vi "NGTS_Create Tasks from Channel Table.vi"(6 "Task Auto Cleanup?":bool, 7 "Physical Address Col (0)":i32, 8 "error in":errorcluster, 9 "Type of IO":enum16{"AI", "AO", "DI", "DO"}(ring), 11 "Channels Properties Table":string[][](array[string])) -> (0 "error out":errorcluster, 2 "List of Devices":string[](array[string]), 3 "DAQmx Task Array Out":refnum<k21>[](array[refnum]))   [LabVIEW 2018]
doc: "Creates DAQmx Tasks based on how many unique chassis IDs there are in the Channel Address column of the Channels Properties Tables. Optionally sets the Auto Cleanup of the tasks when application execution ends.\n\n2007-11 Mike Ashe\nmichael.ashe@imaginatics.net\nCell: 860-961-0876"
uses:
  <userlib>/_OpenG.lib/array/array.llb/Remove Duplicates from 1D Array (String)__ogtk.vi
panel:
  # ". . ."
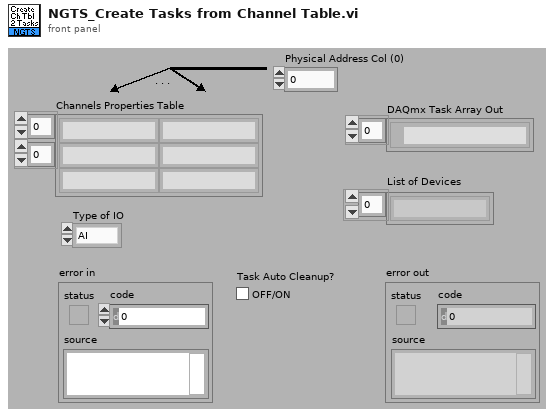
[diagram p1: front panel]
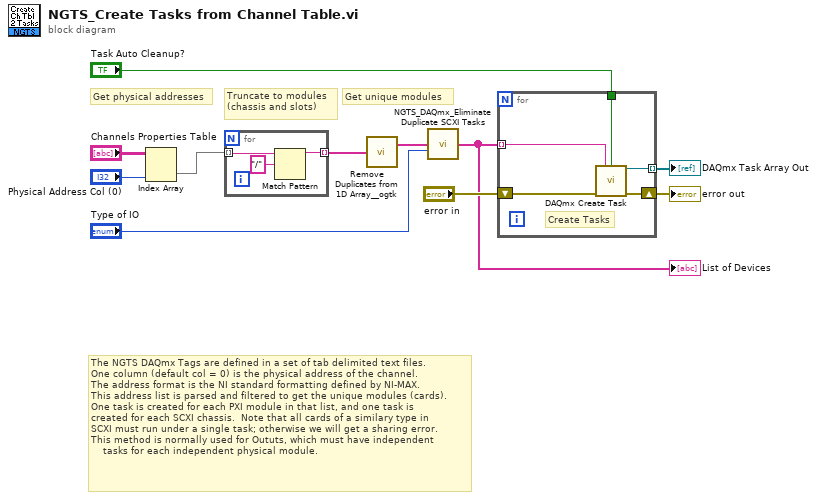
[diagram p0: block diagram]
diagram:
  # "The NGTS DAQmx Tags are defined in a set of tab delimited text files.\nOne column (default col = 0) is the physical address of the channel.\nThe address format is the NI standard formatting defined by NI-MAX.\nThis address list is parsed and filtered to get the unique modules (cards).\nOne task is created for each PXI module in that list, and one task is\ncreated for each SCXI chassis.  Note that all cards of a similary type in\nSCXI must run under a single task; otherwise we will get a sharing error.\nThis method is normally used for Oututs, which must have independent\n    tasks for each independent physical module."
  # "Get unique modules"
  # "Truncate to modules\n(chassis and slots)"
  # "Get physical addresses"
  n1 = Index Array(array="Channels Properties Table", index (col)="Physical Address Col (0)") -> (element=w9:string[])  [unwired: 1 in]
  n2 = for {
    tunnel: w9 -> [w14] mode=indexing
    tunnel: [w12] -> w8 mode=indexing
    n3 = Match Pattern(string=w14, regular expression="/") -> (before substring=w12:string)  [unwired: 1 in, 3 out]
  }
  n4 = call-poly <userlib>:"Remove Duplicates from 1D Array__ogtk.vi"("Input Array"=w8) -> ("Output Array"=w3:string[])  [unwired: 1 out]
  n5 = call "NGTS_DAQmx_Eliminate Duplicate SCXI Tasks.vi"("Tasknames In"=w3, "Type of IO"="Type of IO") -> ("Filtered Tasknames Out"=w1:string[])  [unwired: 13 in]
  "List of Devices" <- w1
  n6 = for {
    tunnel: [w19] -> w7 mode=indexing
    shift-right: [w18] -> w5
    shift-left: "error in" -> [w17]
    tunnel: w1 -> [w15] mode=indexing
    tunnel: "Task Auto Cleanup?" -> [w16]
    # "Create Tasks"
    n7 = call <vilib>:"DAQmx Create Task.vi"("new task name"=w15, "auto cleanup"=w16, "error in"=w17) -> ("task out"=w19:refnum<k21>, "error out"=w18:errorcluster)  [unwired: 11 in]
  }
  "DAQmx Task Array Out" <- w7
  "error out" <- w5
